vi "Get Internal Dir.vi"(0 "VISA resource name":refnum<visa-resource-name>, 5 "Path (\"\")":string, 11 "error in (no error)":errorcluster) -> (4 "VISA resource name out":refnum<visa-resource-name>, 6 "File Name":string[](array[string]), 10 "File Size(KB)":string[](array[string]), 14 "Date Time":timestamp[](array[timestamp]) format="%<%H:%M:%S\n%x>T", 15 "error out":errorcluster)   [LabVIEW 2020, in "Yokogawa GX Series.lvlib"]
doc: "Gets the file list in the internal memory of specified Data Type."
uses:
  <instrlib>/Yokogawa GX Series/Yokogawa GX Series.lvlib
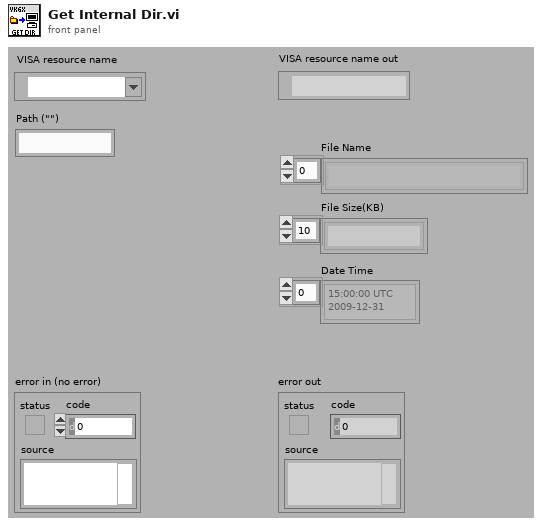
[diagram p1: front panel]
types:
  T1 = typedef "LVDateTimeRec.ctl" = cluster{"fractional second":dbl, "second":i32, "minute":i32, "hour":i32, "day of month":i32, "month":i32, "year":i32, "day of week":i32, "day of year":i32, "DST":i32}
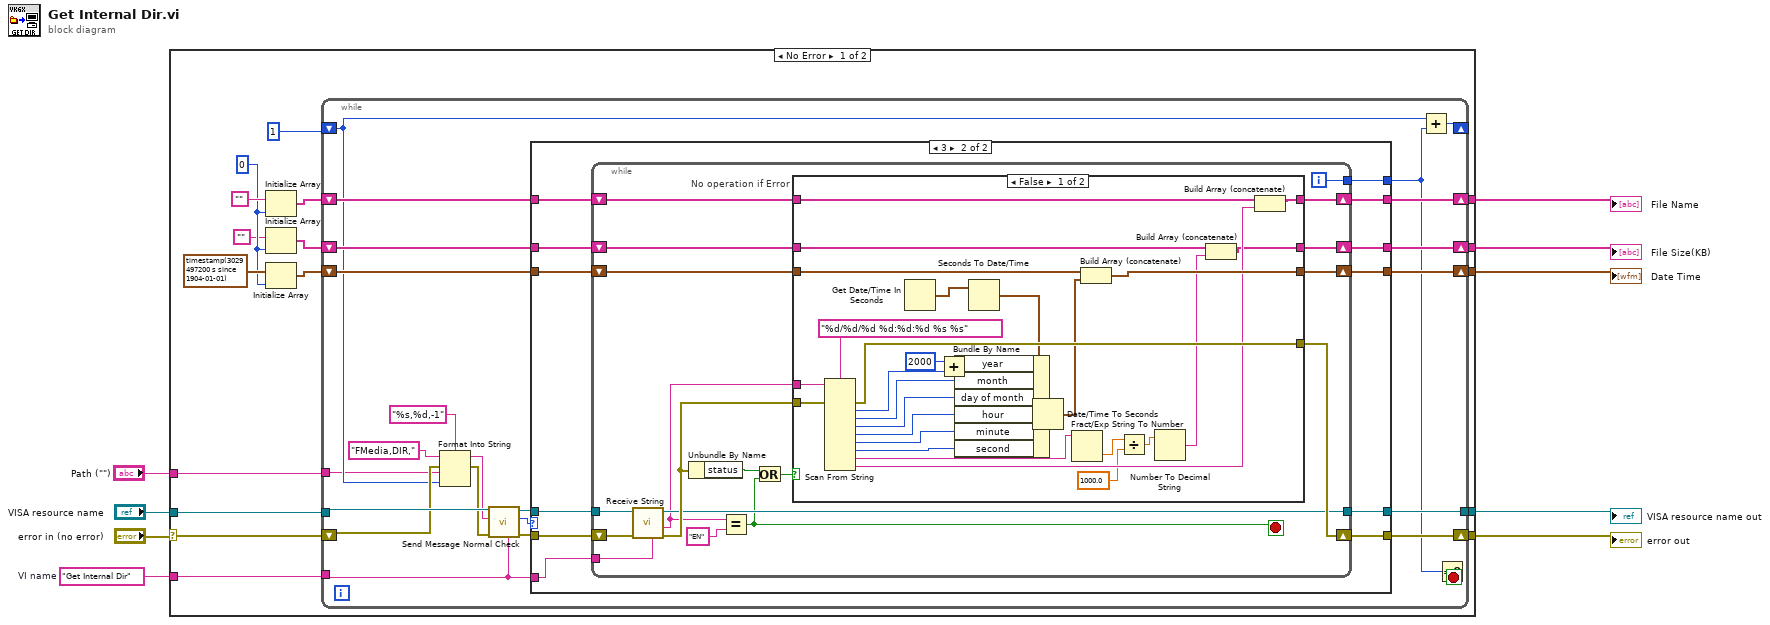
[diagram p0: block diagram]
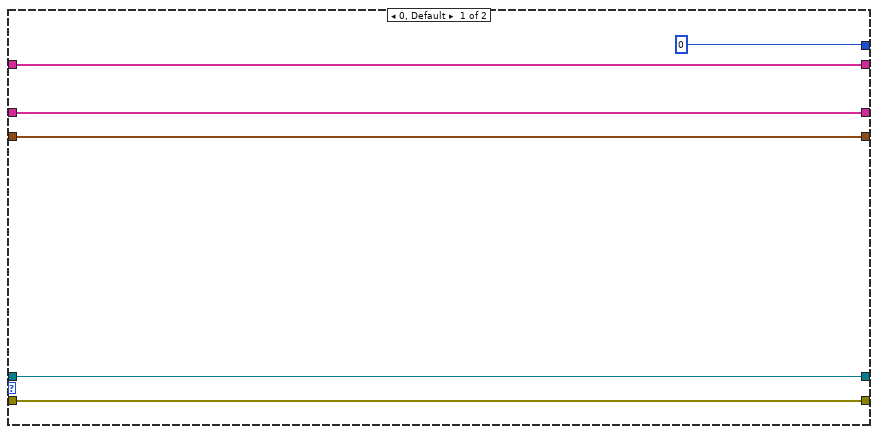
[diagram p2: hidden frame]
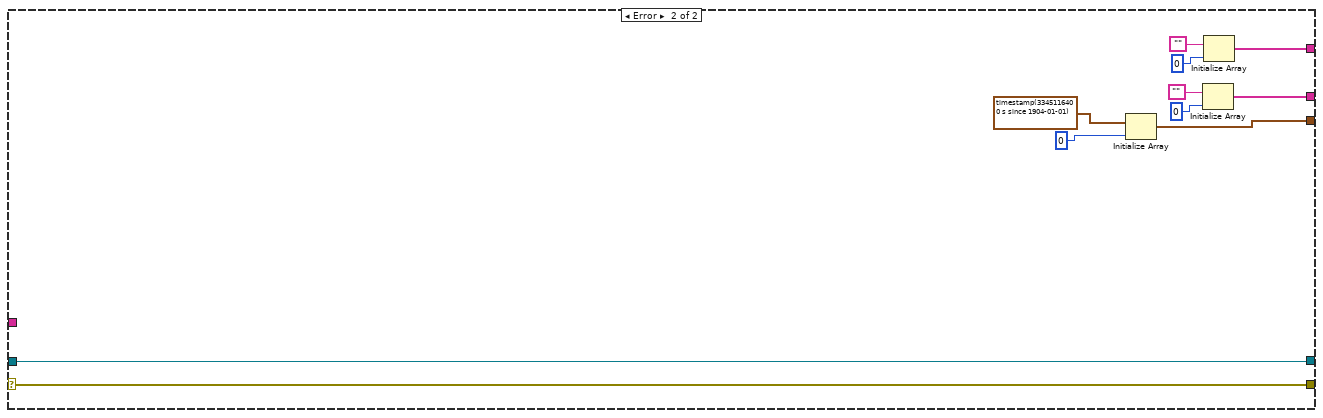
[diagram p4: hidden frame]
diagram:
  w4 = "Get Internal Dir"  # VI name
  n1 = case shown="No Error" "error in (no error)" {
    selector: "error in (no error)" -> [w10 w127]
    tunnel: [w26 w128] -> w9
    tunnel: [w25 w127] -> w8
    tunnel: [w24 w124] -> w7
    tunnel: [w23 w121] -> w6
    tunnel: [w22 w120] -> w5
    tunnel: w4 -> [w14 _]
    tunnel: "VISA resource name" -> [w13 w128]
    tunnel: "Path (\"\")" -> [w12 _]
    frame No Error {
      w16 = 0
      n2 = Initialize Array("" ("File Name"), w16) -> (w20:string[])
      n3 = Initialize Array("", w16) -> (w19:string[])
      n4 = Initialize Array(timestamp(3029497200 s since 1904-01-01) ("Timestamp"), w16) -> (w18:timestamp[])
      n5 = while {
        shift-right: [w47] -> w25
        shift-left: w10 -> [w36]
        shift-right: [w48] -> w22
        shift-left: w18 -> [w49]
        tunnel: w14 -> [w33]
        shift-right: [w44] -> w24
        shift-left: w20 -> [w45]
        shift-right: [w42] -> w23
        shift-left: w19 -> [w43]
        tunnel: [w46] -> w26
        tunnel: w13 -> [w40]
        tunnel: w12 -> [w27]
        shift-right: [w32] -> _
        shift-left: 1 -> [w29]
        stop <- w31 stop-if-true
        n6 = Format Into String(format string="%s,%d,-1", initial string="FMedia,DIR,", error in=w36, w27, w29) -> (resulting string=w34:string, error out=w35:errorcluster)
        n7 = call <instrlib>:"Send Message Normal Check.vi"("Source (\"\")"=w33, "error in (no error)"=w35, "Send Message (\"\")"=w34, "VISA resource name"=w40) -> ("error out"=w41:errorcluster, "Response Type"=w28:i32, "VISA resource name out"=w39:refnum<visa-resource-name>)  [unwired: 2 in, 3 out]
        n8 = case shown="3" w28 {
          tunnel: w49 -> [w53 w67]
          tunnel: [w53 w66] -> w48
          tunnel: [w50 w65] -> w47
          tunnel: [w51 w64] -> w46
          tunnel: w45 -> [w55 w63]
          tunnel: [w55 w62] -> w44
          tunnel: w43 -> [w54 w61]
          tunnel: [w54 w60] -> w42
          tunnel: w41 -> [w50 w56]
          tunnel: w39 -> [w51 w57]
          tunnel: w33 -> [_ w59]
          tunnel: [0 w58] -> w30
          frame 0, Default {
          }
          frame 3 {
            n9 = while {
              tunnel: w59 -> [w68]
              tunnel: [w79] -> w64
              tunnel: w57 -> [w73]
              tunnel: [w70] -> w58
              shift-right: [w77] -> w62
              shift-left: w63 -> [w78]
              shift-right: [w75] -> w60
              shift-left: w61 -> [w76]
              shift-right: [w83] -> w66
              shift-left: w67 -> [w84]
              shift-right: [w82] -> w65
              shift-left: w56 -> [w74]
              i -> [w70]
              stop <- w69 stop-if-true
              n10 = call <instrlib>:"Receive String.vi"("Source (\"\")"=w68, "error in (no error)"=w74, "VISA resource name"=w73) -> ("error out"=w85:errorcluster, "Read Buffer"=w71:string, "VISA resource name out"=w79:refnum<visa-resource-name>)  [unwired: 1 in, 5 out]
              n11 = Unbundle By Name(w85) -> ("status"=w81:bool)
              n12 = Equal?(x=w71, y="EN") -> (x = y?=w69:bool)
              n13 = Or(x=w81, y=w69) -> (x .or. y?=w80:bool)
              n14 = case "No operation if Error" shown="False" w80 {
                tunnel: w71 -> [w112 _]
                tunnel: [w111 w117] -> w83
                tunnel: w85 -> [w110 w114]
                tunnel: [w109 w114] -> w82
                tunnel: w84 -> [w97 w117]
                tunnel: w78 -> [w101 w116]
                tunnel: [w100 w116] -> w77
                tunnel: w76 -> [w92 w115]
                tunnel: [w91 w115] -> w75
                frame False {
                  n15 = Scan From String(format string="%d/%d/%d %d:%d:%d %s %s", input string=w112, error in=w110) -> (error out=w109:errorcluster, output 1=w107:i32, output 2=w106:i32, output 3=w105:i32, output 4=w104:i32, output 5=w103:i32, output 6=w102:i32, output 7=w87:string, output 8=w99:string)  [unwired: 1 in, 10 out]
                  n16 = Get Date/Time In Seconds() -> (seconds since 1Jan1904=w94:timestamp)
                  n17 = Add(x=2000, y=w107) -> (x+y=w96:i32)
                  n18 = Seconds To Date/Time(time stamp (now)=w94) -> (date time rec=w108:T1)  [unwired: 1 in]
                  n19 = Bundle By Name(cluster=w108, "year"=w96, "month"=w106, "day of month"=w105, "hour"=w104, "minute"=w103, "second"=w102) -> (w93:T1)
                  n20 = Date/Time To Seconds(2:w93) -> (0:w98:timestamp)  [unwired: 1 in]
                  n21 = Fract/Exp String To Number(string=w87) -> (number=w86:dbl)  [unwired: 3 in, 1 out]
                  n22 = Build Array (concatenate)(w97, w98) -> (w111:timestamp[])
                  n23 = Divide ("商")(x=w86, y=1000.0) -> (x/y=w89:dbl)
                  n24 = Number To Decimal String(number=w89) -> (decimal integer string=w88:string)  [unwired: 1 in]
                  n25 = Build Array (concatenate)(w92, w88) -> (w91:string[])
                  n26 = Build Array (concatenate)(w101, w99) -> (w100:string[])
                }
                frame True {
                }
              }
            }
          }
        }
        n27 = Add(x=w29, y=w30) -> (x+y=w32:i32)
        n28 = Equal To 0?(x=w30) -> (x = 0?=w31:bool)
      }
    }
    frame Error {
      n29 = Initialize Array(timestamp(3345116400 s since 1904-01-01), 0) -> (w120:timestamp[])
      n30 = Initialize Array("", 0) -> (w121:string[])
      n31 = Initialize Array("", 0) -> (w124:string[])
    }
  }
  "error out" <- w8
  "VISA resource name out" <- w9
  "File Name" <- w7
  "File Size(KB)" <- w6
  "Date Time" <- w5
